vi "Define Type.vi"(5 "Type":T1, 7 "Attributes":T2, 10 "Definition":T3, 11 "Type in":refnum<class "Type.lvclass">) -> (3 "Type out":refnum<class "Type.lvclass">)   [LabVIEW 2020, in "Conditu2.lvlib" / "Columns.lvlib" / "Type.lvclass"]
uses:
  Type.lvclass
  Definition.ctl
  Attributes.ctl
  Field Type.ctl
  Type.lvclass/Type.ctl
  Conditu2.lvlib
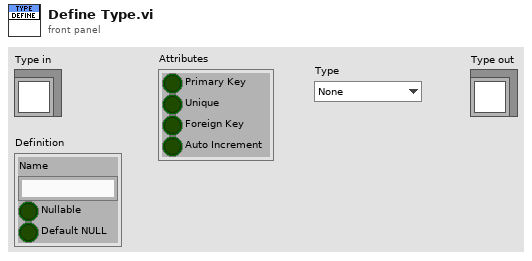
[diagram p1: front panel]
types:
  T1 = typedef "Conditu2.lvlib/Field Type.ctl" = enum16{"None", "ID", "Boolean", "Integer", "Double", "Timestamp", "String", "Text", "Entity"}
  T2 = typedef "Conditu2.lvlib/Attributes.ctl" = cluster{"Primary Key":bool, "Unique":bool, "Foreign Key":bool, "Auto Increment":bool}
  T3 = typedef "Conditu2.lvlib/Columns.lvlib/Type.lvclass/Definition.ctl" = cluster{"Name":string, "Nullable":bool, "Default NULL":bool}
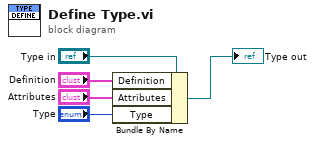
[diagram p0: block diagram]
diagram:
  n1 = Bundle By Name(cluster="Type in", "Definition"="Definition", "Attributes"="Attributes", "Type"="Type") -> (→"Type out":refnum<class "Type.lvclass">)
